vi "Fast Holo1 SLM.vi"   [LabVIEW 2014]
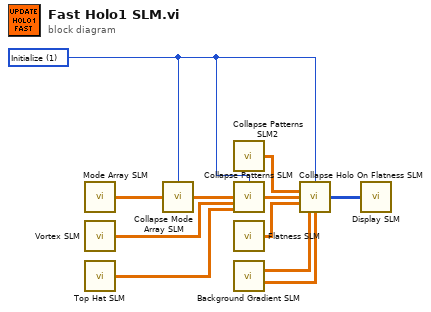
[diagram p0: block diagram]
diagram:
  w11 = u16 1 items=["Read", "Initialize"] ("Action")
  n1 = call "Mode Array SLM.vi"() -> ("mode array"=w4:dbl[][][])  [unwired: 15 in]
  n2 = call "Vortex SLM.vi"() -> ("Vortex"=w7:dbl[][])  [unwired: 15 in]
  n3 = call "Top Hat SLM.vi"() -> ("Top hat"=w8:dbl[][])  [unwired: 15 in]
  n4 = call "Collapse Mode Array SLM.vi"("Action"=w11, "mode array"=w4) -> ("collapsed mode array"=w5:dbl[][])  [unwired: 13 in]
  n5 = call "Collapse Patterns SLM2.vi"() -> ("collapsed patterns"=w3:dbl[][])  [unwired: 15 in]
  n6 = call "Collapse Patterns SLM.vi"("Action"=w11, "collapsed mode array"=w5, "Vortex"=w7, "Top hat"=w8) -> ("collapsed patterns"=w6:dbl[][])  [unwired: 11 in]
  n7 = call "Flatness SLM.vi"() -> ("flatness"=w9:dbl[][])  [unwired: 15 in]
  n8 = call "Background Gradient SLM.vi"() -> ("gradient"=w2:dbl[][], "holo mask"=w1:dbl[][])  [unwired: 14 in]
  n9 = call "Collapse Holo On Flatness SLM.vi"("Action"=w11, "collapsed patterns 2"=w3, "collapsed patterns"=w6, "flatness"=w9, "gradient"=w2, "holo mask"=w1) -> ("displayed matrix"=w10:u8[][])  [unwired: 9 in]
  n10 = call "Display SLM.vi"("displayed matrix"=w10) -> ()  [unwired: 14 in, 1 out]
